vi "Sample Transfer Get Source and Target Samples.vi"(8 "error in (no error)":errorcluster, 11 "cRIO-CO2 in":refnum<class "cRIO-CO2.lvclass">) -> (0 "error out":errorcluster, 1 "Sample in Target Container":refnum<class "Sample.lvclass">, 2 "Sample in Source Container":refnum<class "Sample.lvclass">, 3 "cRIO-CO2 out":refnum<class "cRIO-CO2.lvclass">)   [LabVIEW 2015, in "cRIO-Carbondioxide.lvlib" / "cRIO-CO2.lvlib" / "cRIO-CO2.lvclass"]
uses:
  cRIO-CO2.lvclass
  subs/Sample/Sample.lvclass
  cRIO-CO2.lvclass/cRIO-CO2.ctl
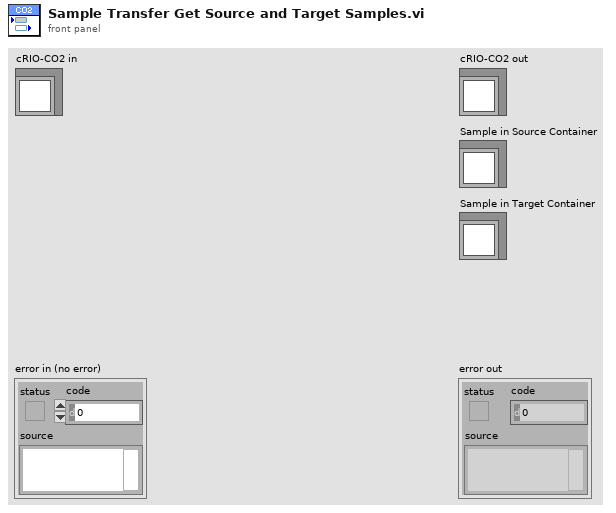
[diagram p1: front panel]
types:
  T1 = typedef "Sample Transfer Container Enumerator.ctl" = enum16{"None", "Sample 1", "Sample 2", "Sample 3", "Sample 4", "Sample 5", "Storage 01", "Storage 02", "Storage 03", "Storage 04", "Storage 05", "Storage 06", "Storage 07", "Storage 08", "Storage 09", "Storage 10", "Storage 11", "Storage 12", "Syringe", "Undefined"}
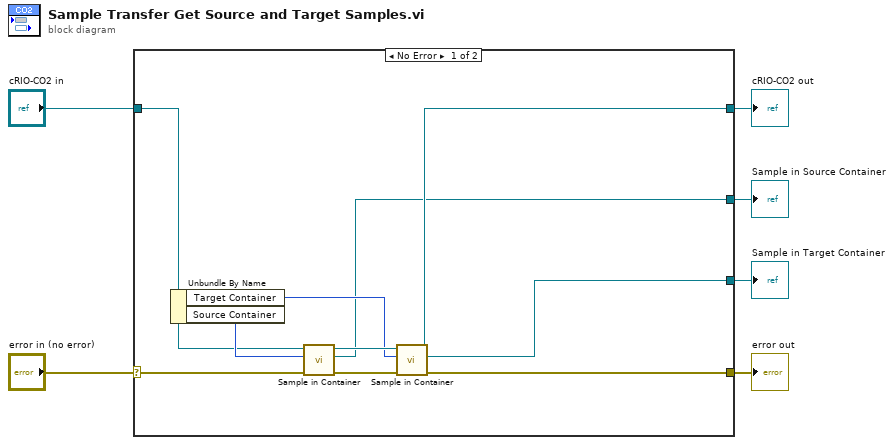
[diagram p0: block diagram]
diagram:
  n1 = case shown="No Error" "error in (no error)" {
    selector: "error in (no error)" -> [w16 w18]
    tunnel: [w9 w18] -> w5
    tunnel: [w10 w17] -> w3
    tunnel: "cRIO-CO2 in" -> [w11 w17]
    tunnel: [w8 _] -> w2
    tunnel: [w7 _] -> w1
    frame No Error {
      n2 = Unbundle By Name(w11) -> ("Target Container"=w12:T1, "Source Container"=w15:T1)
      n3 = call "Sample in Container.vi"("error in (no error)"=w16, "Container"=w15, "cRIO-CO2 in"=w11) -> ("error out"=w14:errorcluster, "Sample"=w8:refnum<class "Sample.lvclass">, "cRIO-CO2 out"=w13:refnum<class "cRIO-CO2.lvclass">)  [unwired: 6 in]
      n4 = call "Sample in Container.vi"("error in (no error)"=w14, "Container"=w12, "cRIO-CO2 in"=w13) -> ("error out"=w9:errorcluster, "Sample"=w7:refnum<class "Sample.lvclass">, "cRIO-CO2 out"=w10:refnum<class "cRIO-CO2.lvclass">)  [unwired: 6 in]
    }
    frame Error {
    }
  }
  "error out" <- w5
  "cRIO-CO2 out" <- w3
  "Sample in Source Container" <- w2
  "Sample in Target Container" <- w1
